vi "Test Log Debug Message.vi"(8 "error in (no error)":errorcluster, 11 "Test Case In":refnum<class "Logger Test.lvclass">) -> (0 "error out":errorcluster, 3 "Test Case Out":refnum<class "Logger Test.lvclass">)   [LabVIEW 2020, in "Logger Test.lvclass"]
uses:
  Logger Test.lvclass
  source/Framework Test Suite/Mock Process/Mock Process.lvclass
  C:/Git/astemes-triarc-framework/source/Framework/Process/Process.lvclass
  C:/Git/astemes-triarc-framework/source/Framework/Logging/Logging.lvclass
  source/Framework Test Suite/Mock Log Handler/Mock Log Handler.lvclass
  source/Framework/Process/Process.lvclass/Process.ctl
  <vilib>/Astemes/LUnit/Test Case.lvclass/Test Case.ctl
  28fd62af-8587-454a-b2c4-b3331bc08afc.vi
  5169cdc5-36c4-4e58-91ce-5d6a482ec58f.vi
  10d72d36-b88f-466e-832e-0ad287d19119.vi
  source/Framework/Process/Public/Lifecycle/Get Lifecycle State.vi
  source/Framework/Process/Protected/Messaging/Send Message.vi
  <vilib>/Astemes/LUnit/Palette/Pass.vi
  <vilib>/Astemes/LUnit/Palette/Fail.vi
  <vilib>/Astemes/LUnit/Compare Variants.vi
  <vilib>/Astemes/LUnit/Describe Comparison.vi
  <vilib>/Astemes/LUnit/Set Assertion Type.vi
  <vilib>/Utility/error.llb/Clear Errors.vi
  source/Framework/Process/Private/SubVIs/Handle Debug Data.vi
  <vilib>/Astemes/LUnit/Add test result.vi
  <vilib>/Astemes/LUnit/Variant to string.vi
  <vilib>/AdvancedString/1D String Array to Delimited String.vi
  <vilib>/Utility/High Resolution Relative Seconds.vi
  <vilib>/Astemes/LUnit/LUnit Record Assertion Result.vi
  <vilib>/Astemes/LUnit/LUnit Aggregate Assertion Results.vi
  <vilib>/Astemes/LUnit/Method Result/LUnit Merge Status.vi
  <vilib>/Astemes/LUnit/LUnit Concatenate result strings.vi
  <vilib>/Utility/error.llb/Error Cluster From Error Code.vi
  source/Framework/Process/Public/Read Name.vi
  <vilib>/Utility/Data Type/Get Type Information.vi
  <vilib>/Utility/LVClass/Get LV Class Name.vi
  source/Framework/Logging/Logging.lvclass
  Logger Test.lvclass/Logger Test.ctl
  source/Framework/Process/Process.lvclass
  C:/Git/astemes-triarc-framework/source/Framework/Base/Base.lvclass
  C:/Git/astemes-triarc-framework/source/Framework/Configuration File/Configuration File.lvclass
  C:/Git/astemes-triarc-framework/source/Framework/Configuration/Configuration.lvclass
  C:/Git/astemes-triarc-framework/source/Framework/Error Handler Interface/Error Handler Interface.lvclass
  C:/Git/astemes-triarc-framework/source/Framework Test Suite/Mock Process/Mock Process.lvclass
  C:/Git/astemes-triarc-framework/source/Framework/Async Handler/Async Handler.lvclass
  C:/Git/astemes-triarc-framework/source/Framework/Helper Loop/Helper Loop.lvclass
  <vilib>/Astemes/LUnit/Test Case.lvclass
  C:/Git/astemes-triarc-framework/source/Framework Test Suite/Mock Log Handler/Mock Log Handler.lvclass
  C:/Program Files (x86)/National Instruments/LabVIEW 2020/vi.lib/Astemes/LUnit/Test Case.lvclass
  C:/Git/astemes-triarc-framework/tests/Logger Test/Logger Test.lvclass
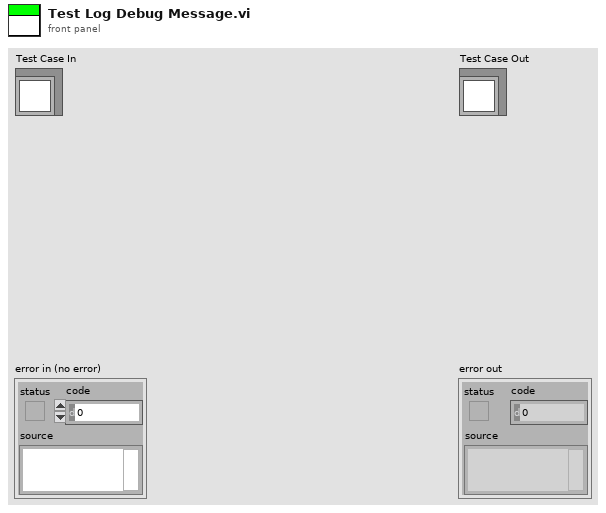
[diagram p1: front panel]
types:
  T1 = typedef "Mock Log Handler.lvclass/Log Entry.ctl" = cluster{"Level":string, "Source":string, "Message":string}
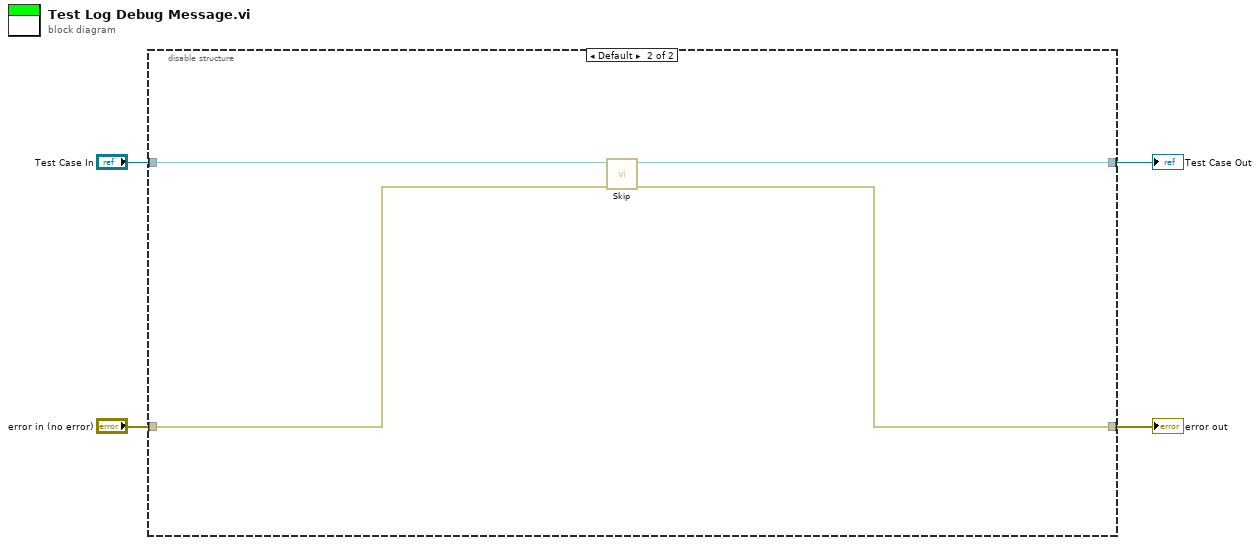
[diagram p0: block diagram]
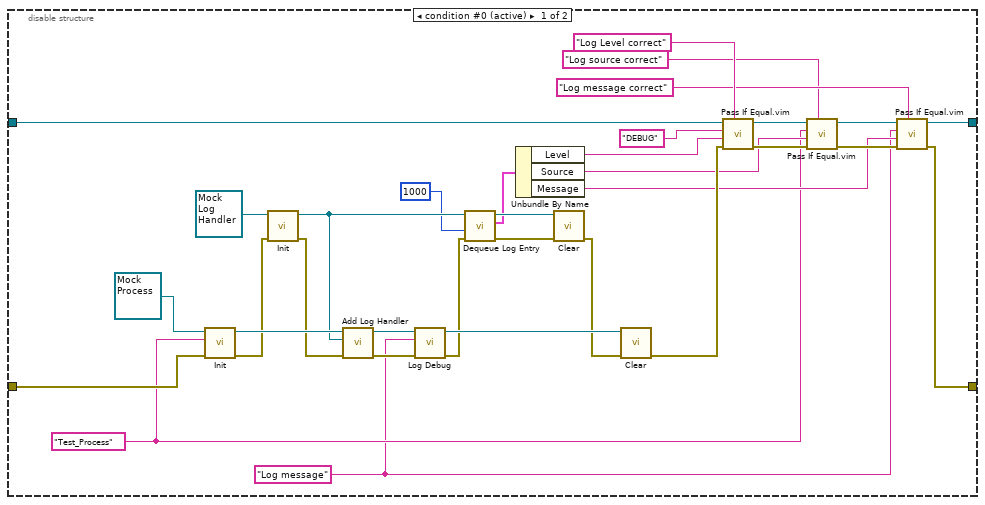
[diagram p2: hidden frame]
diagram:
  n1 = disable-structure shown="Default" {
    disable-tunnel: "Test Case In" -> [w37 w39]
    disable-tunnel: "error in (no error)" -> [w31 w41]
    disable-tunnel: [w15 w38] -> w2
    disable-tunnel: [w11 w40] -> w1
    frame condition #0 (active) {
      w5 = "Log message" ("Message")
      w6 = "Test_Process" ("Name")
      n2 = call-dynamic "Init.vi"("error in (no error)"=w31, "Name"=w6, "Mock Process In"=refnum<class "Mock Process.lvclass"> refnum) -> ("error out"=w29:errorcluster, "Mock Process Out"=w34:refnum<class "Mock Process.lvclass">)  [unwired: 7 in]
      n3 = call-dynamic "Init.vi"("error in (no error)"=w29, "Mock Log Handler In"=refnum<class "Mock Log Handler.lvclass"> refnum ("Mock Log Handler.lvclass")) -> ("error out"=w28:errorcluster, "Mock Log Handler Out"=w25:refnum<class "Mock Log Handler.lvclass">)  [unwired: 8 in]
      n4 = call "Add Log Handler.vi"("error in (no error)"=w28, "Log Handler"=w25, "Process In"=w34) -> ("error out"=w33:errorcluster, "Process Out"=w23:refnum<class "Mock Process.lvclass">)  [unwired: 7 in]
      n5 = call "Log Debug.vi"("error in (no error)"=w33, "Message"=w5, "Logging In"=w23) -> ("error out"=w21:errorcluster, "Logging Out"=w22:refnum<class "Mock Process.lvclass">)  [unwired: 7 in]
      n6 = call "Dequeue Log Entry.vi"("error in (no error)"=w21, "timeout in ms (-1)"=1000, "Mock Log Handler in"=w25) -> ("error out"=w26:errorcluster, "Entry"=w19:T1, "Mock Log Handler out"=w27:refnum<class "Mock Log Handler.lvclass">)  [unwired: 5 in, 1 out]
      n7 = Unbundle By Name(w19) -> ("Level"=w18:string, "Source"=w8:string, "Message"=w7:string)
      n8 = call-dynamic "Clear.vi"("error in (no error)"=w26, "Mock Log Handler In"=w27) -> ("error out"=w20:errorcluster)  [unwired: 9 in]
      n9 = call-dynamic "Clear.vi"("error in (no error)"=w20, "Mock Process In"=w22) -> ("error out"=w12:errorcluster)  [unwired: 9 in]
      n10 = call "Pass If Equal.vim"("Description"="Log Level correct", "error in (no error)"=w12, "Actual"=w18, "Expected"="DEBUG", "LUnit Test Case In"=w37) -> ("error out"=w14:errorcluster, "LUnit Test Case Out"=w36:refnum<class "Logger Test.lvclass">)  [unwired: 5 in]
      n11 = call "Pass If Equal.vim"("Description"="Log source correct", "error in (no error)"=w14, "Actual"=w8, "Expected"=w6, "LUnit Test Case In"=w36) -> ("error out"=w13:errorcluster, "LUnit Test Case Out"=w16:refnum<class "Logger Test.lvclass">)  [unwired: 5 in]
      n12 = call "Pass If Equal.vim"("Description"="Log message correct", "error in (no error)"=w13, "Actual"=w7, "Expected"=w5, "LUnit Test Case In"=w16) -> ("error out"=w11:errorcluster, "LUnit Test Case Out"=w15:refnum<class "Logger Test.lvclass">)  [unwired: 5 in]
    }
    frame condition #1 {
      n13 = call <vilib>:"Skip.vi"("error in (no error)"=w41, "LUnit Test Case In"=w39) -> ("error out"=w40:errorcluster, "LUnit Test Case Out"=w38:refnum<class "Logger Test.lvclass">)  [unwired: 8 in]
    }
  }
  "error out" <- w1
  "Test Case Out" <- w2
